vi "Calculate Throttle Values.vi"(8 "error in (no error)":errorcluster, 11 "RDS Helm Actor in":refnum<class "RDS Helm Actor.lvclass">) -> (0 "error out":errorcluster, 3 "RDS Helm Actor out":refnum<class "RDS Helm Actor.lvclass">)   [LabVIEW 2015, in "RDS Helm Actor.lvlib" / "RDS Helm Actor.lvclass"]
uses:
  Actors/RDS Helm Actor/RDS Helm Actor/RDS Helm Actor.lvclass
  Actors/RDS Helm Actor/RDS Helm Actor/RDS Helm Actor.lvclass/RDS Helm Actor.ctl
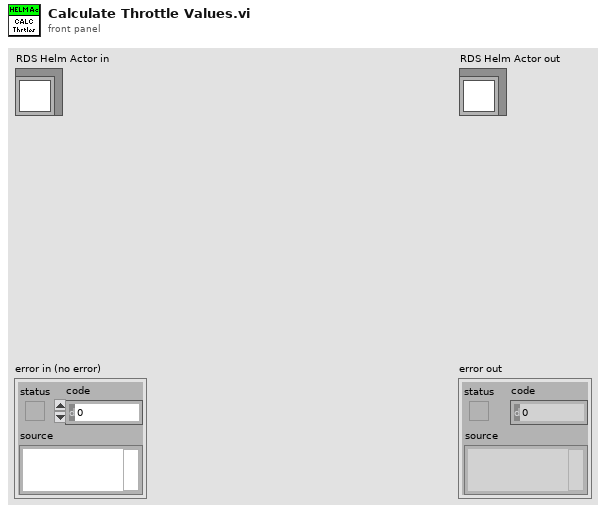
[diagram p1: front panel]
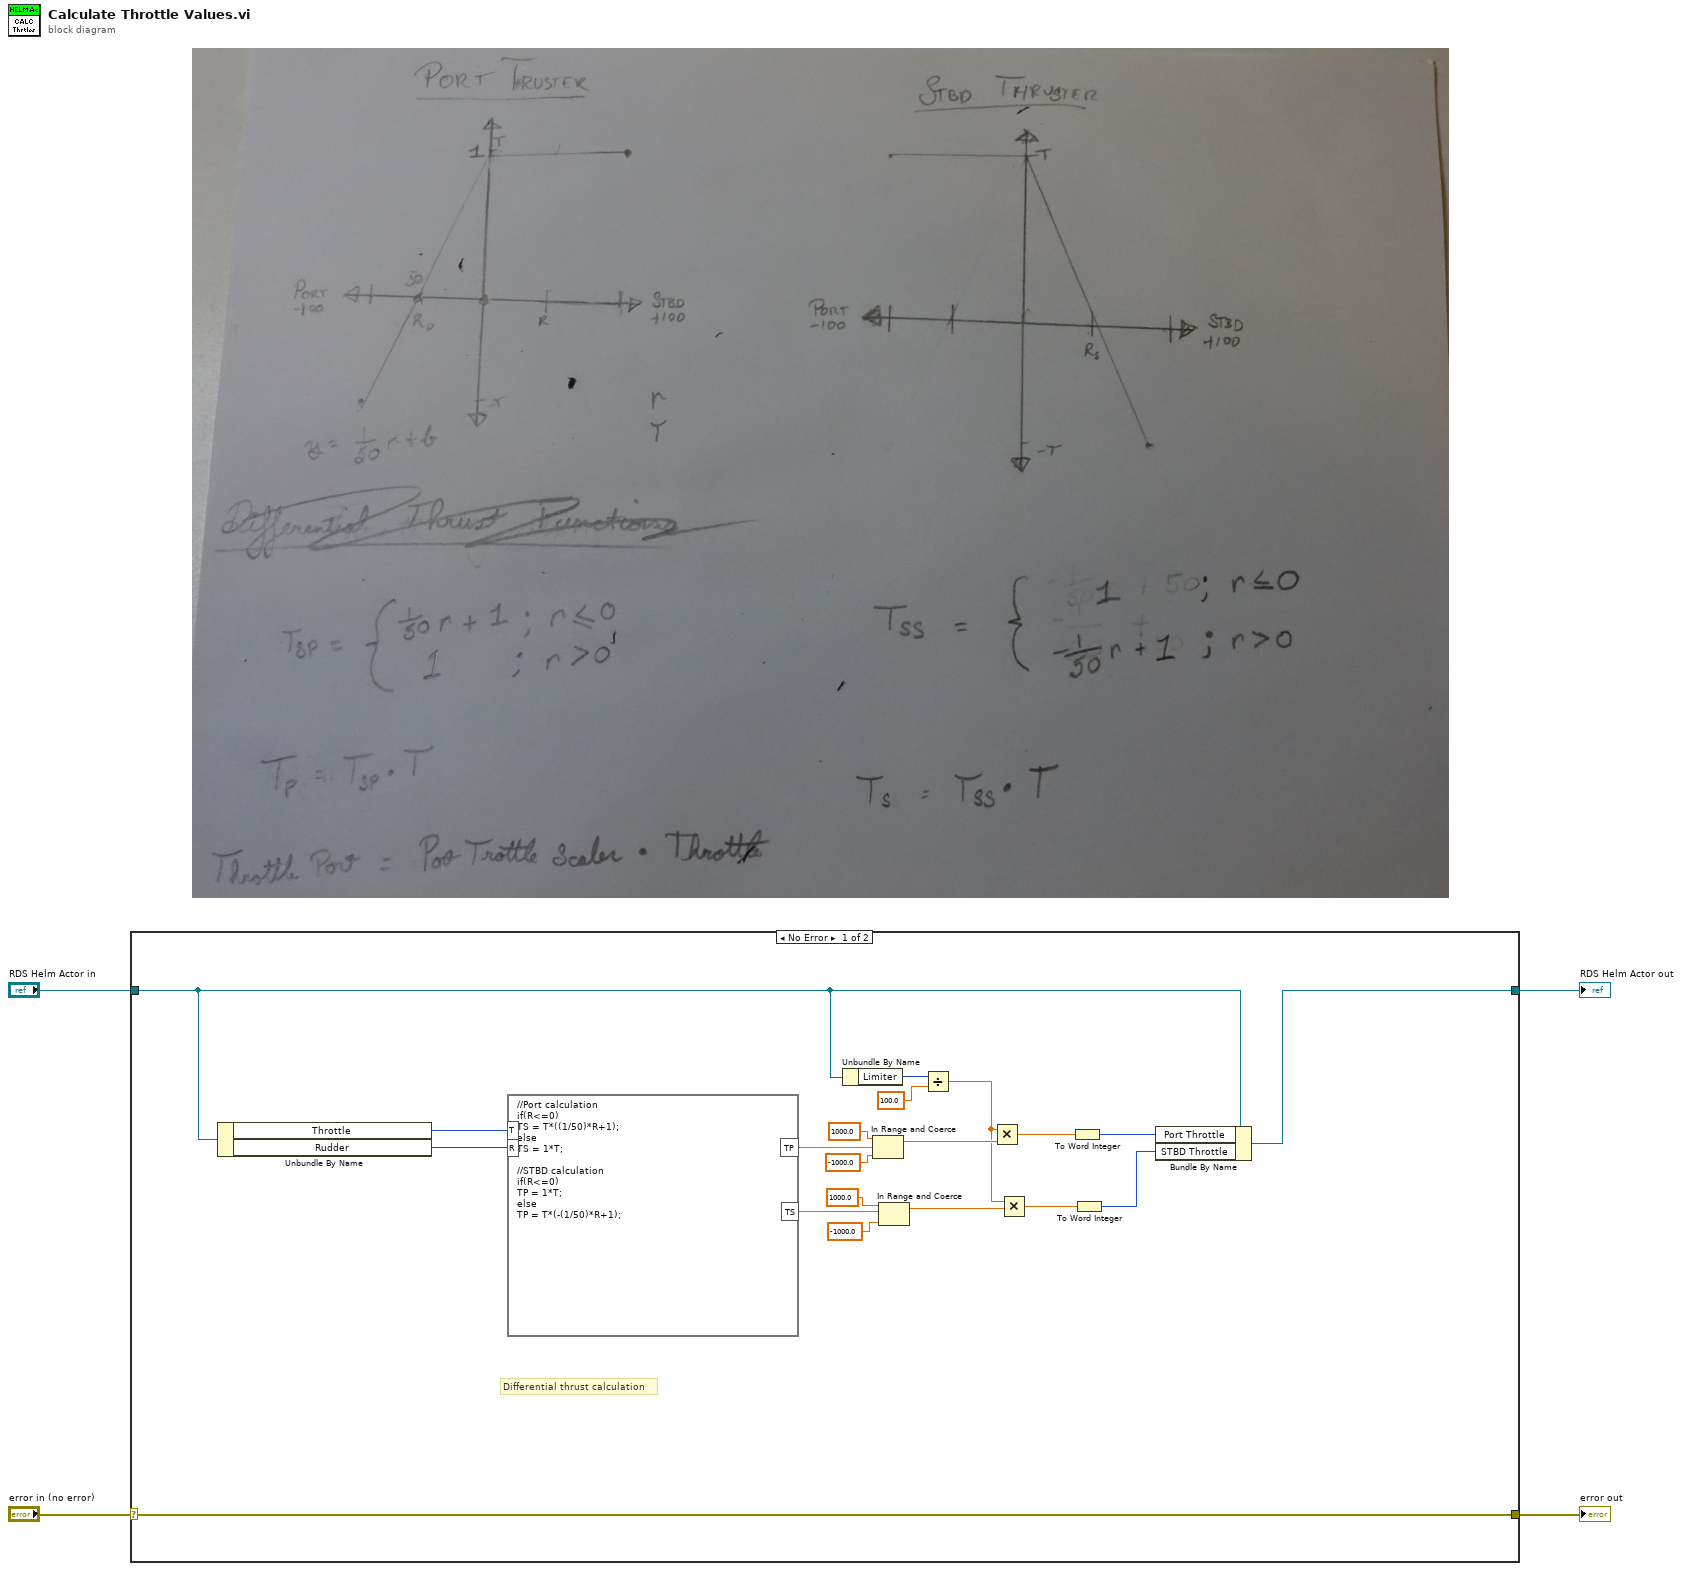
[diagram p0: block diagram]
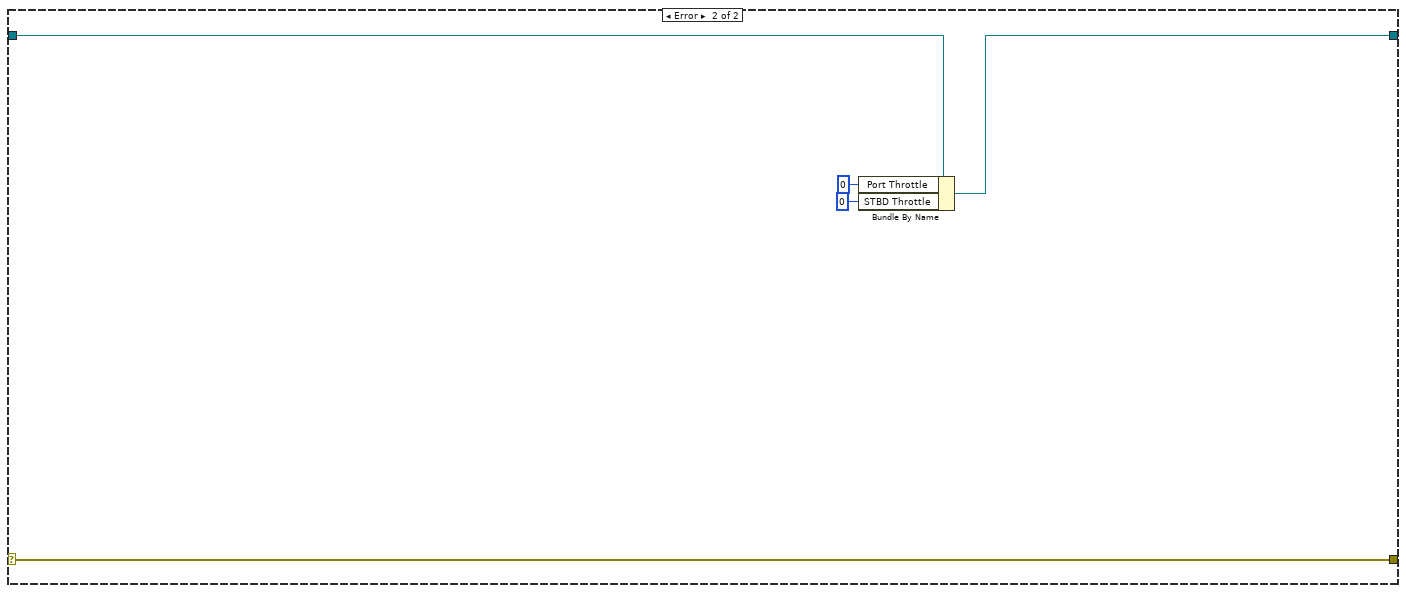
[diagram p2: hidden frame]
diagram:
  n1 = case shown="No Error" "error in (no error)" {
    selector: "error in (no error)" -> [w24 w29]
    tunnel: [w24 w29] -> w3
    tunnel: [w15 w27] -> w1
    tunnel: "RDS Helm Actor in" -> [w13 w28]
    frame No Error {
      # "Differential thrust calculation"
      n2 = Unbundle By Name(w13) -> ("Throttle"=w23:i16, "Rudder"=w22:i8)
      n3 = formula code="//Port calculation\nif(R<=0)\nTS = T*((1/50)*R+1); \nelse\nTS = 1*T;\n\n//STBD calculation\nif(R<=0)\nTP = 1*T;\nelse\nTP = T*(-(1/50)*R+1);"("R"=w22, "T"=w23) -> ("TP"=w21:dbl, "TS"=w16:dbl)
      n4 = Unbundle By Name(w13) -> ("Limiter"=w12:u8)
      n5 = In Range and Coerce(upper limit=1000.0, x=w21, lower limit=-1000.0) -> (coerced(x)=w14:dbl)  [unwired: 1 out]
      n6 = In Range and Coerce(upper limit=1000.0, x=w16, lower limit=-1000.0) -> (coerced(x)=w10:dbl)  [unwired: 1 out]
      n7 = Divide(x=w12, y=100.0) -> (x/y=w9:dbl)
      n8 = Multiply(x=w9, y=w14) -> (x*y=w6:dbl)
      n9 = Multiply(x=w9, y=w10) -> (x*y=w8:dbl)
      n10 = To Word Integer(number=w6) -> (16bit integer=w5:i16)
      n11 = To Word Integer(number=w8) -> (16bit integer=w7:i16)
      n12 = Bundle By Name(cluster=w13, "Port Throttle"=w5, "STBD Throttle"=w7) -> (w15:refnum<class "RDS Helm Actor.lvclass">)
    }
    frame Error {
      n13 = Bundle By Name(cluster=w28, "Port Throttle"=i16 0, "STBD Throttle"=i16 0) -> (w27:refnum<class "RDS Helm Actor.lvclass">)
    }
  }
  "error out" <- w3
  "RDS Helm Actor out" <- w1
